vi "Mod_OFDM_Write_Waveform_To_File.VI"(0 "Complex Waveform":T2={"t0"=0.0, "dt"=1.0, "Y"=[]} {"Y" format="%.3f"; "dt" format="%^.2e"; "t0" format="%.4f"}, 2 "Configuration in":variant, 11 "error IO":errorcluster, 13 "Config_Waveform":T1={"Phase Continous \nWaveform"=FALSE, "Store Waveform\nTo a File"=FALSE, "Generate Waveform"=TRUE, "Store Waveform + \nConfiguration To Files"=FALSE}) -> (4 "Complex Waveform":T2={"t0"=0.0, "dt"=1.0, "Y"=[]} {"Y" format="%.3f"; "dt" format="%^.2e"; "t0" format="%.4f"}, 15 "error out":errorcluster)   [LabVIEW 2010]
doc: "The VI stores the complex waveform generated for the OFDM frame. The waveform is stored in a Datalog file alongwith the configuration information. The configuration information is stored to retrieve the OFDM Frame summary for which the the waveform is generated.\n\nThe waveform can be read back by the \"Mod_OFDM_Read_Waveform_From_File\" VI."
uses:
  <vilib>/addons/Modulation/Analog/controls/Complex Data Waveform.ctl
  <vilib>/Waveform/WDTFileIO.llb/ Write Waveforms to File (1D).vi
panel:
  in  "all waveforms \nin record":waveform(dbl)[](array[waveform])
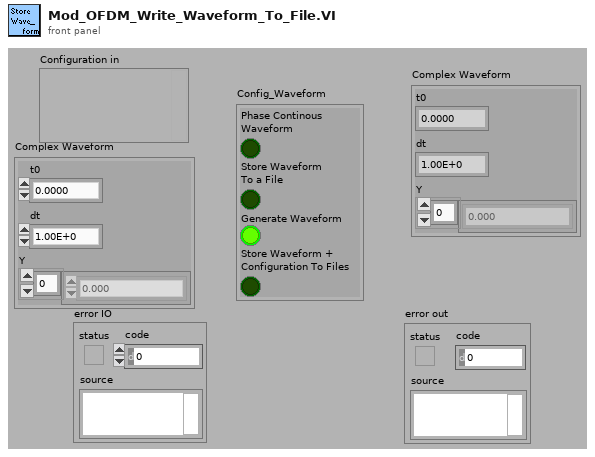
[diagram p1: front panel]
types:
  T1 = cluster{"Phase Continous \nWaveform":bool, "Store Waveform\nTo a File":bool, "Generate Waveform":bool, "Store Waveform + \nConfiguration To Files":bool}
  T2 = typedef "Complex Data Waveform.ctl" = cluster{"t0":dbl, "dt":dbl, "Y":cdb[]}
  T3 = enum16{"open", "open or create", "create or replace", "create", "open (read only)"}
  T4 = enum32{"existing file", "new file", "new or existing file", "existing dir", "new dir", "new or existing dir", "existing file (use LLBs)", "new file (use LLBs)", "new or existing file (use LLBs)", "new or existing file or directory (use LLBs)"}
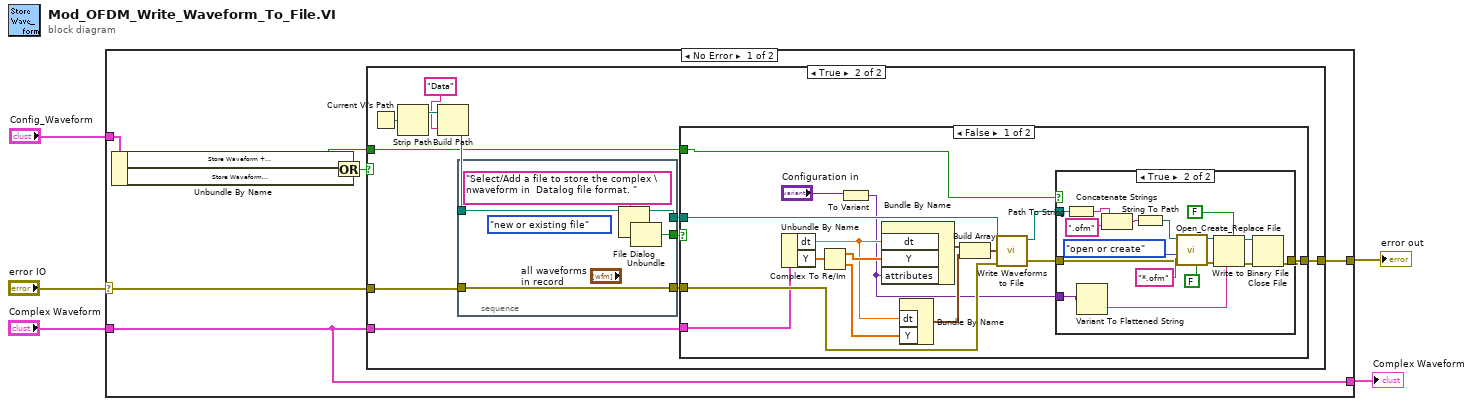
[diagram p0: block diagram]
diagram:
  n1 = case shown="No Error" "error IO" {
    selector: "error IO" -> [w12 w66]
    tunnel: "Complex Waveform" -> [w10 _]
    tunnel: [w11 w66] -> w3
    tunnel: [w10 _] -> w2
    tunnel: "Config_Waveform" -> [w9 _]
    frame No Error {
      n2 = Unbundle By Name(w9) -> ("Store Waveform + \nConfiguration To Files"=w6:bool, "Store Waveform\nTo a File"=w8:bool)
      n3 = Or(x=w6, y=w8) -> (x .or. y?=w7:bool)
      n4 = case shown="True" w7 {
        tunnel: w12 -> [w13 w20]
        tunnel: [w13 w17] -> w11
        tunnel: w10 -> [_ w16]
        tunnel: w6 -> [_ w14]
        frame False {
        }
        frame True {
          n5 = Current VI's Path() -> (path=w24:path)
          n6 = Strip Path(path=w24) -> (stripped path=w23:path)  [unwired: 1 out]
          n7 = Build Path(base path=w23, name or relative path="Data") -> (appended path=w21:path)
          n8 = stacked-sequence {
            tunnel: w21 -> [w65]
            tunnel: [w64] -> w19
            tunnel: w20 -> [w64]
            tunnel: [w63] -> w18
            tunnel: [w62] -> w15
            frame #0 {
              (unwired) T4."new or existing file" ("select mode (2)")
              n9 = File Dialog(7:"Select/Add a file to store the complex \nwaveform in  Datalog file format. " ("prompt"), 11:w65) -> (0:w60:errorcluster, 1:w62:bool, 3:w63:path)  [unwired: 5 in, 1 out]
              n10 = Unbundle(w60) -> ()  [unwired: 3 out]
            }
          }
          n11 = case shown="False" w15 {
            tunnel: w19 -> [w35 w59]
            tunnel: w18 -> [w30 _]
            tunnel: [w32 w59] -> w17
            tunnel: w16 -> [w34 _]
            tunnel: w14 -> [w31 _]
            frame False {
              n12 = Unbundle By Name(w34) -> ("dt"=w27:dbl, "Y"=w40:cdb[])
              n13 = Complex To Re/Im(x + iy=w40) -> (x=w28:dbl[], y=w39:dbl[])
              n14 = To Variant(anything="Configuration in") -> (Variant=w25:variant)
              n15 = Bundle By Name("dt"=w27, "Y"=w28, "attributes"=w25) -> (w38:waveform(dbl))  [unwired: 1 in]
              n16 = Bundle By Name("dt"=w27, "Y"=w39) -> (w37:waveform(dbl))  [unwired: 1 in]
              n17 = Build Array(w38, w37) -> (w36:waveform(dbl)[])
              n18 = call-poly <vilib>:"Write Waveforms to File.vi"("error in (no error)"=w35, "waveform array"=w36, "file path (dialog if empty)"=w30) -> ("error out"=w33:errorcluster, "new file path (Not A Path if cancelled)"=w29:path)  [unwired: 7 in]
              n19 = case shown="True" w31 {
                tunnel: w33 -> [w41 w57]
                tunnel: [w41 w53] -> w32
                tunnel: w29 -> [_ w50]
                tunnel: w25 -> [_ w44]
                frame False {
                }
                frame True {
                  n20 = Path To String(path=w50) -> (string=w49:string)
                  n21 = Variant To Flattened String(Variant=w44) -> (data string=w43:string)  [unwired: 1 out]
                  n22 = Concatenate Strings(w49, ".ofm" ("pattern")) -> (w46:string)
                  n23 = String To Path(string=w46) -> (path=w47:path)
                  n24 = call <vilib>:"Open_Create_Replace File.vi"("advisory dialog? (display:T)"=FALSE, "default name"="*.ofm", "error in (no error)"=w57, "function (open:0)"=T3."open or create", "file path"=w47) -> ("error out"=w56:errorcluster, "refnum"=w51:refnum<file>)  [unwired: 3 in, 2 out]
                  n25 = Write to Binary File(file (use dialog)=w51, data=w43, error in=w56, 5:FALSE ("prepend array or string size? (T)")) -> (refnum out=w54:refnum<file>, error out=w55:errorcluster)  [unwired: 2 in, 1 out]
                  n26 = Close File(refnum=w54, error in=w55) -> (error out=w53:errorcluster)  [unwired: 1 out]
                }
              }
            }
            frame True {
            }
          }
        }
      }
    }
    frame Error {
    }
  }
  "error out" <- w3
  "Complex Waveform" <- w2
